vi "chart set table.vi"(8 "error in (no error)":errorcluster, 11 "chart":u32) -> (0 "error out":errorcluster)   [LabVIEW 2015, in "xlsxwriter.lvlib"]
doc: "void chart_set_table(lxw_chart chart);"
uses:
  xlsxwriter.lvlib
  xlsxwriter.dll
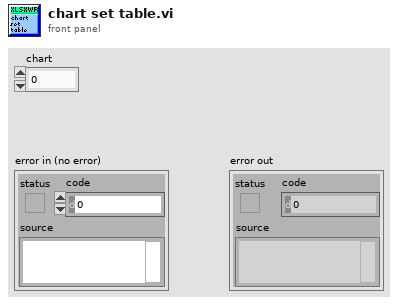
[diagram p1: front panel]
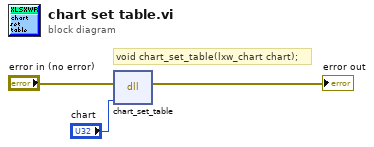
[diagram p0: block diagram]
diagram:
  # "void chart_set_table(lxw_chart chart);"
  n1 = dll-call lib="C:/Users/WDAGUtilityAccount/Desktop/lv_vis_added_cell/xlsxwriter.*" fn="chart_set_table"(error in="error in (no error)", "chart"="chart") -> (error out=→"error out":errorcluster)  [unwired: 4 in, 1 out]
